vi "Replace Subset Element.vi"(2 "error in (no error)":errorcluster, 3 "new element/subarray":refnum<class "Generic Plugin.lvclass">, 4 "index":i32, 5 "Controller Array in":refnum<class "Controller Array.lvclass">) -> (0 "error out":errorcluster, 1 "Controller Array out":refnum<class "Controller Array.lvclass">)   [LabVIEW 2020, in "RxnRover.lvlib" / "Controller Array.lvclass"]
uses:
  Controller Array.lvclass
  Controller/Generic Plugin.lvclass
  Controller Array.lvclass/Controller Array.ctl
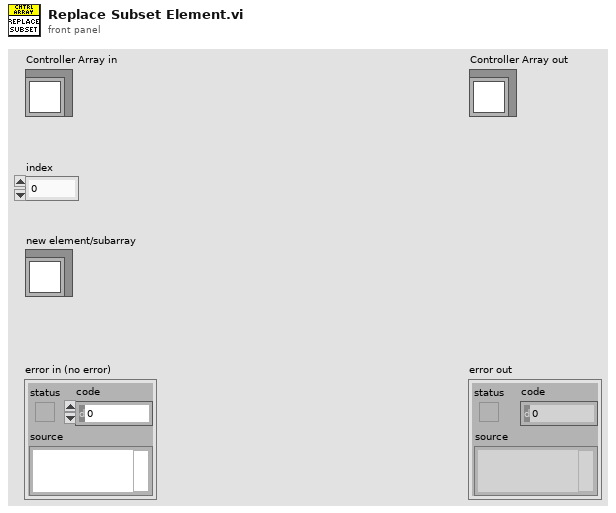
[diagram p1: front panel]
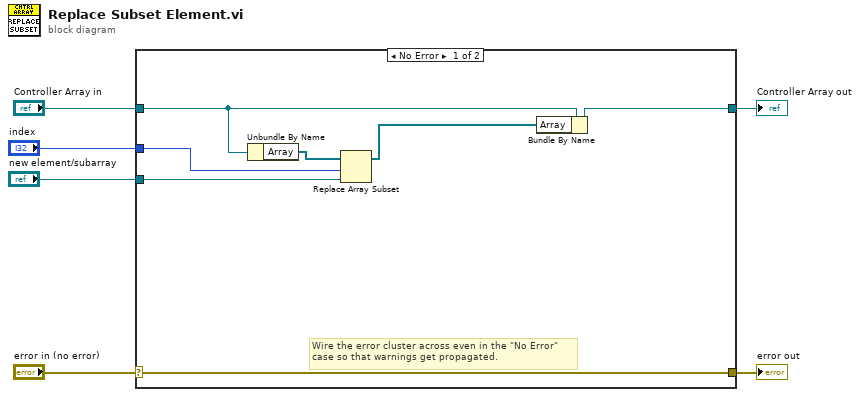
[diagram p0: block diagram]
diagram:
  n1 = case shown="No Error" "error in (no error)" {
    selector: "error in (no error)" -> [w13 w15]
    tunnel: [w13 w15] -> w5
    tunnel: [w8 w14] -> w3
    tunnel: "Controller Array in" -> [w12 w14]
    tunnel: "new element/subarray" -> [w10 _]
    tunnel: "index" -> [w9 _]
    frame No Error {
      # "Wire the error cluster across even in the \"No Error\"\ncase so that warnings get propagated."
      n2 = Unbundle By Name(w12) -> ("Array"=w11:refnum<class "Generic Plugin.lvclass">[])
      n3 = Replace Array Subset(array=w11, new element=w10, index=w9) -> (w7:refnum<class "Generic Plugin.lvclass">[])
      n4 = Bundle By Name(cluster=w12, "Array"=w7) -> (w8:refnum<class "Controller Array.lvclass">)
    }
    frame Error {
    }
  }
  "error out" <- w5
  "Controller Array out" <- w3
